vi "Calculate Bone Vectors.vi"() -> ()   [LabVIEW 2011, in "KinectOne.lvlib"]
doc: "This example demonstrates how to calculate vectors between two joints ('bones') and calculate the angle between two 'bone' vectors."
uses:
  vi.lib/MakerHub/KinectOne/KinectOne.lvlib
  vi.lib/MakerHub/KinectOne/Private/Type Defs/JointType.ctl
  vi.lib/MakerHub/KinectOne/Private/Initialize Image [Color].vi
  vi.lib/MakerHub/KinectOne/Private/kinectRead [BodyFrame].vi
  Microsoft.Kinect
  C:/github/makerhub/KinectOne/LabVIEW/vi.lib/MakerHub/KinectOne/Private/Libs/BodyFrameDataInterface.dll
  vi.lib/MakerHub/KinectOne/Private/Libs/BodyFrameDataInterface.dll
panel:
  out "Angle Between Bones (deg)":dbl=nan
  out "Joint 1-2 Vector":dbl[](array[numeric])
  out "Joint 2-3 Vector":dbl[](array[numeric])
  in  "Joints":T2={"Joint 1"=enum."ShoulderRight", "Joint 2"=enum."ElbowRight", "Joint 3"=enum."HandRight"}
  out "Body Index Image":T3(plugin-control)
  in  "Stop Button":bool
  # "Calculate Bone Vectors Example\n\nThis example demonstrates how to calculate 'bone' vectors based on joint positions.\n\n1. Make sure you have the Kinect SDK 2.0 installed.\n2. Connect the Kinect sensor to the computer via USB.\n3. Click the Run button.\n4. Stand in front of the Kinect sensor.\n\nHave feedback or need help?  Visit the MakerHub forums at www.labviewmakerhub.com/forums/kinectone"
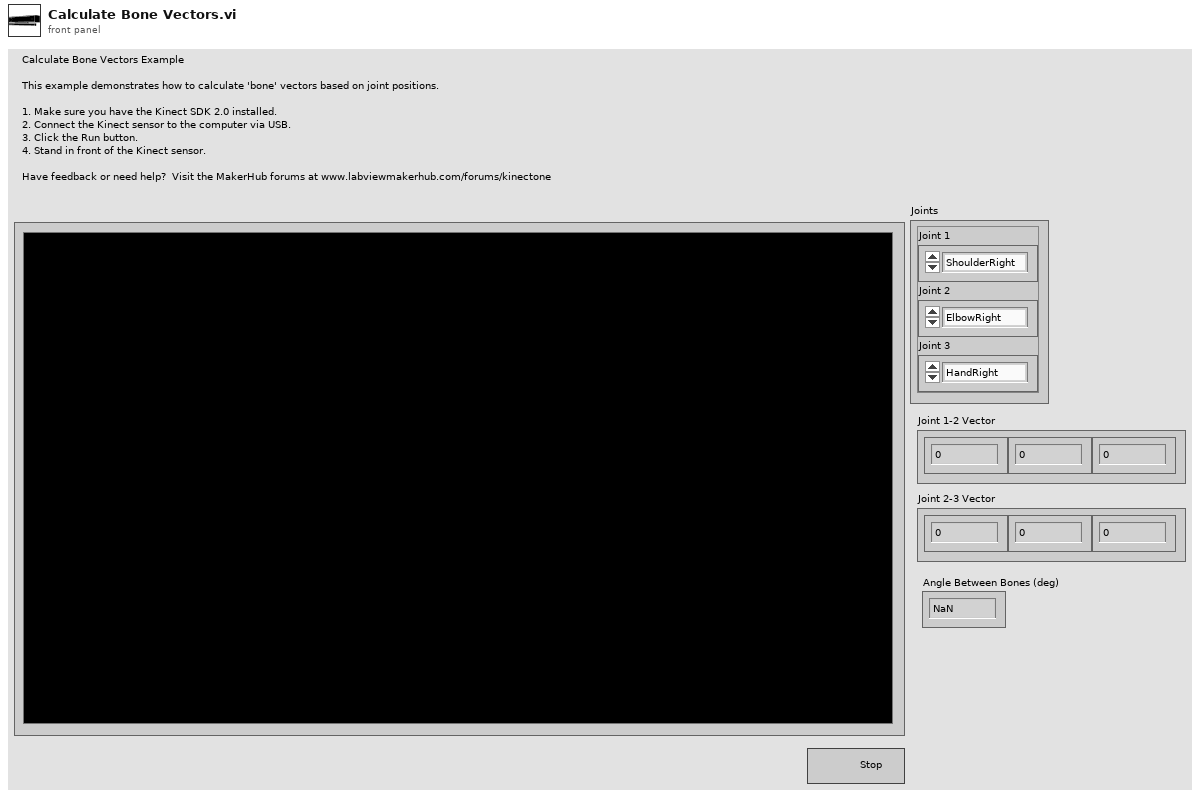
[diagram p1: front panel]
types:
  T1 = typedef "KinectOne.lvlib/JointType.ctl" = enum16{"SpineBase", "SpineMid", "Neck", "Head", "ShoulderLeft", "ElbowLeft", "WristLeft", "HandLeft", "ShoulderRight", "ElbowRight", "WristRight", "HandRight", "HipLeft", "KneeLeft", "AnkleLeft", "FootLeft", "HipRight", "KneeRight", "AnkleRight", "FootRight", "SpineShoulder", "HandTipLeft", "ThumbLeft", "HandTipRight", "ThumbRight"}
  T2 = cluster{"Joint 1":T1, "Joint 2":T1, "Joint 3":T1}
  T3 = typedef "IMAQ Image.ctl" = refnum<image>
  T4 = typedef "KinectOne.lvlib/KinectSensor References.ctl" = cluster{"KinectSensor":refnum<k24>, "MultiSourceFrameReader":refnum<k24>, "BodyFrameDataInterface":refnum<k24>}
  T5 = typedef "KinectOne.lvlib/BodyData.ctl" = cluster{"ClippedEdges":T6, "HandLeftConfidence":T7, "HandLeftState":T8, "HandRightConfidence":T9, "HandRightState":T10, "IsRestricted":bool, "IsTracked":bool, "JointOrientations":refnum<k24>, "Joints":refnum<k24>, "Lean":refnum<k24>, "LeanTrackingState":T11, "TrackingId":u64}
  T6 = typedef "KinectOne.lvlib/ClippedEdges.ctl" = enum16{"None", "Right", "Left", "Top", "Bottom"}
  T7 = typedef "KinectOne.lvlib/HandLeftConfidence.ctl" = enum16{"Low", "High"}
  T8 = typedef "KinectOne.lvlib/HandLeftState.ctl" = enum16{"Unknown", "NotTracked", "Open", "Closed", "Lasso"}
  T9 = typedef "KinectOne.lvlib/HandRightConfidence.ctl" = enum16{"Low", "High"}
  T10 = typedef "KinectOne.lvlib/HandRightState.ctl" = enum16{"Unknown", "NotTracked", "Open", "Closed", "Lasso"}
  T11 = typedef "KinectOne.lvlib/LeanTrackingState.ctl" = enum16{"NotTracked", "Inferred", "Tracked"}
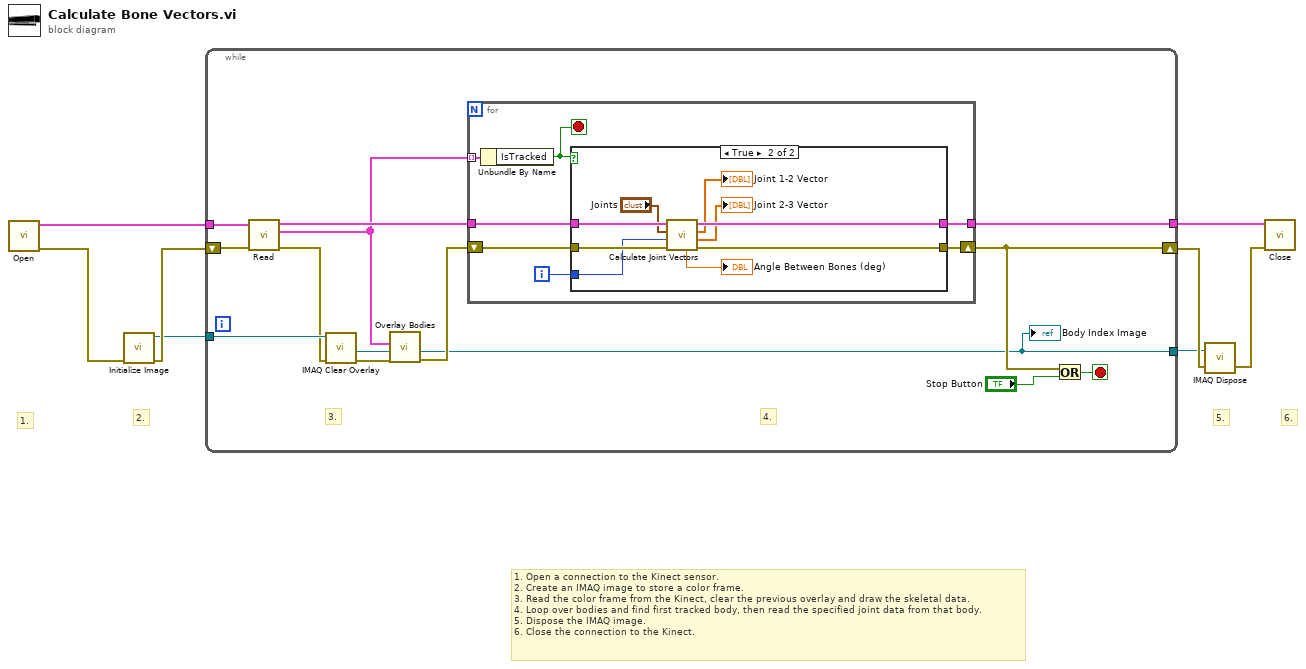
[diagram p0: block diagram]
diagram:
  # "1. Open a connection to the Kinect sensor.\n2. Create an IMAQ image to store a color frame.\n3. Read the color frame from the Kinect, clear the previous overlay and draw the skeletal data.\n4. Loop over bodies and find first tracked body, then read the specified joint data from that body.\n5. Dispose the IMAQ image.\n6. Close the connection to the Kinect."
  # "6."
  # "5."
  # "2."
  # "1."
  n1 = call "Open.vi"() -> ("Error Out"=w7:errorcluster, "KinectSensor References out"=w3:T4)  [unwired: 10 in]
  n2 = call-poly "Initialize Image.vi"("Error In"=w7) -> ("Error Out"=w2:errorcluster, "Color Image"=w1:T3)  [unwired: 9 in]
  n3 = while {
    shift-right: [w14] -> w6
    shift-left: w2 -> [w16]
    tunnel: [w9] -> w5
    tunnel: [w12] -> w4
    tunnel: w3 -> [w13]
    tunnel: w1 -> [w20]
    stop <- w22 stop-if-true
    # "4."
    # "3."
    n4 = call-poly "Read.vi"("error in (no error)"=w16, "KinectSensor References in"=w13) -> ("error out"=w18:errorcluster, "Body Data"=w10:T5[], "KinectSensor References out"=w11:T4)  [unwired: 7 in]
    n5 = call "IMAQ Clear Overlay"("error in (no error)"=w18, "Image"=w20) -> ("error out"=w17:errorcluster, "Image Out"=w19:T3)  [unwired: 8 in]
    n6 = call "Overlay Bodies.vi"("Error In"=w17, "Image"=w19, "Body Data"=w10) -> ("Error Out"=w15:errorcluster, "Image Out"=w9:T3)  [unwired: 7 in]
    "Body Index Image" <- w9
    n7 = for {
      tunnel: [w27] -> w12
      tunnel: w11 -> [w26]
      shift-right: [w28] -> w14
      shift-left: w15 -> [w29]
      tunnel: w10 -> [w25] mode=indexing
      i -> [w23]
      stop <- w24 stop-if-true
      n8 = Unbundle By Name(w25) -> ("IsTracked"=w24:bool)
      n9 = case shown="True" w24 {
        tunnel: w29 -> [w30 w40]
        tunnel: [w30 w32] -> w28
        tunnel: [w31 w39] -> w27
        tunnel: w26 -> [w31 w38]
        tunnel: w23 -> [_ w37]
        frame False {
          # "No Tracked Bodies"
        }
        frame True {
          n10 = call "Calculate Joint Vectors.vi"("Error In"=w40, "Body Index"=w37, "Joints"="Joints", "KinectSensor References"=w38) -> ("Error Out"=w32:errorcluster, "Joint 2-3 Vector"=→"Joint 2-3 Vector":dbl[], "Joint 1-2 Vector"=→"Joint 1-2 Vector":dbl[], "KinectSensor References"=w39:T4, "Angle Between Bones (deg)"=→"Angle Between Bones (deg)":dbl)  [unwired: 3 in]
        }
      }
    }
    n11 = Or(x=w14, y="Stop Button") -> (x .or. y?=w22:bool)
  }
  n12 = call "IMAQ Dispose"("Image"=w5, "error in (no error)"=w6) -> ("error out"=w8:errorcluster)  [unwired: 4 in]
  n13 = call "Close.vi"("Error In"=w8, "KinectSensor References"=w4) -> ()  [unwired: 9 in, 1 out]
